vi "Config Frequency.vi"(8 "error in":errorcluster, 10 "Frequency (1000 Hz)":dbl(ring)=1000.0 items=["50"=50.0, "60"=60.0, "70"=70.0, "80"=80.0, "100"=100.0, "120"=120.0, "140"=140.0, "160"=160.0, "200"=200.0, "240"=240.0, "300"=300.0, "400"=400.0, "500"=500.0, "600"=600.0, "700"=700.0, "800"=800.0, "1000"=1000.0, "1200"=1200.0, "1400"=1400.0, "1600"=1600.0, "2000"=2000.0, "2400"=2400.0, "3000"=3000.0, "4000"=4000.0, "5000"=5000.0, "6000"=6000.0, "7000"=7000.0, "8000"=8000.0, "10000"=10000.0, "12000"=12000.0, "14000"=14000.0, "16000"=16000.0, "20000"=20000.0], 11 "VISA resource name":refnum<visa-resource-name>) -> (0 "error out":errorcluster, 3 "VISA resource name out":refnum<visa-resource-name>)   [LabVIEW 2025]
doc: "This VI sets the test frequency at which measurements are to be taken."
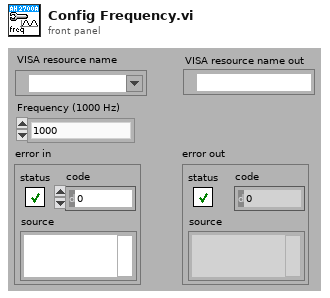
[diagram p1: front panel]
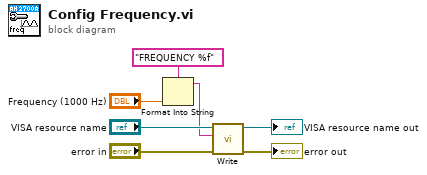
[diagram p0: block diagram]
diagram:
  n1 = Format Into String(format string="FREQUENCY %f", "Frequency (1000 Hz)") -> (resulting string=w6:string)  [unwired: 2 in, 1 out]
  n2 = call "Write.vi"("error in"="error in", "command"=w6, "VISA resource name"="VISA resource name") -> ("error out"=→"error out":errorcluster, "VISA resource name out"=→"VISA resource name out":refnum<visa-resource-name>)  [unwired: 7 in]
